vi "LoginVI.vi"() -> ()   [LabVIEW 2017]
uses:
  NameSurnameID.vi
panel:
  in  "Login information":T1
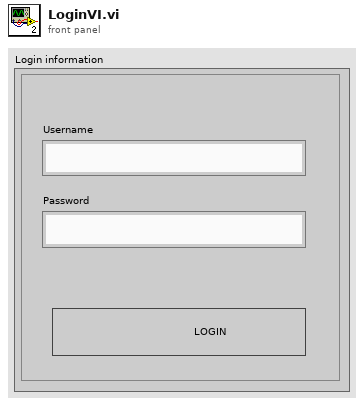
[diagram p1: front panel]
types:
  T1 = cluster{"Username":string, "Password":string, "Login button":bool}
  T2 = enum32{"Invalid", "Standard", "Closed", "Hidden", "Minimized", "Maximized"}
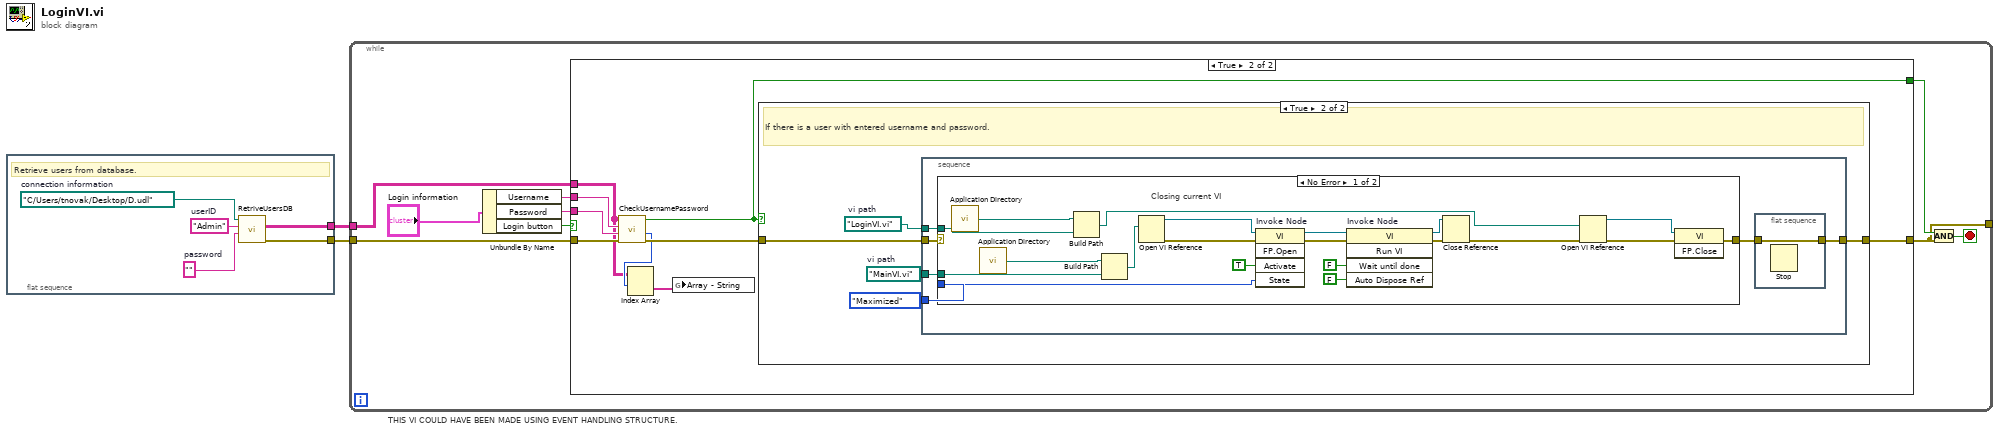
[diagram p0: block diagram]
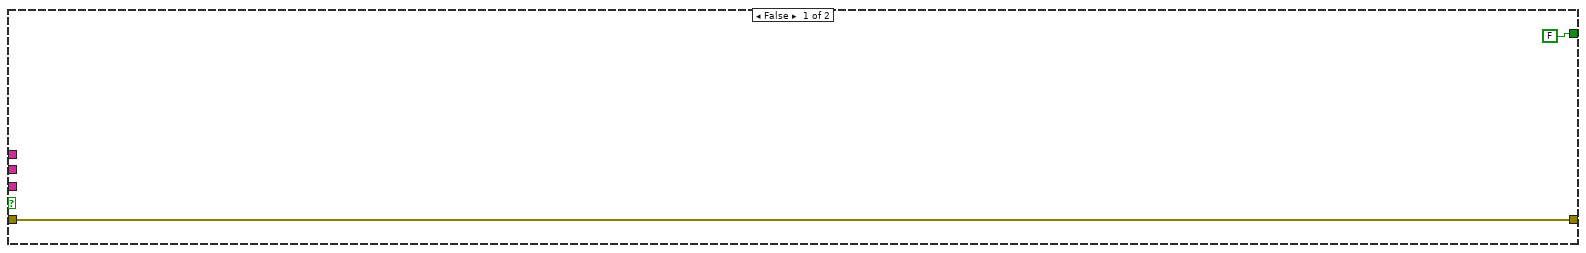
[diagram p2: hidden frame]
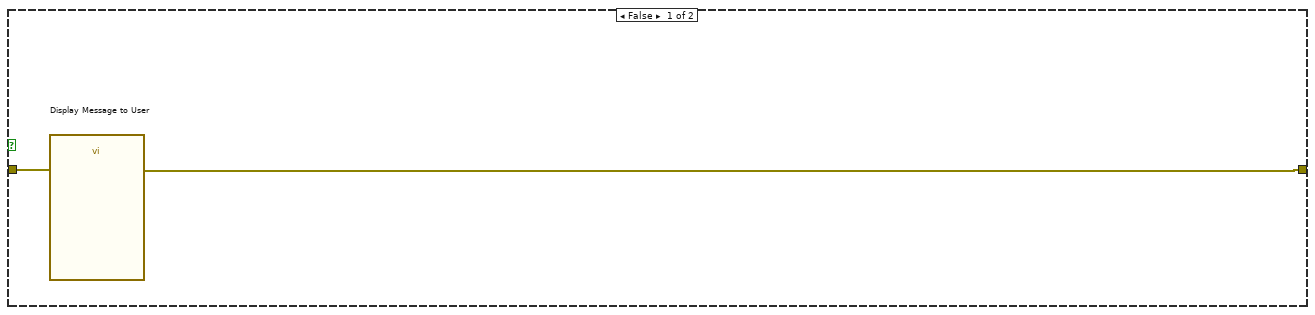
[diagram p3: hidden frame]
diagram:
  # "THIS VI COULD HAVE BEEN MADE USING EVENT HANDLING STRUCTURE."
  n1 = flat-sequence {
    tunnel: [w4] -> w2
    tunnel: [w3] -> w1
    frame #0 {
      w5 = ""  # password
      w6 = "Admin"  # userID
      w7 = path "C:/Users/tnovak/Desktop/D.udl"  # connection information
      # "Retrieve users from database."
      n2 = call "RetriveUsersDB.vi"("password"=w5, "userID"=w6, "connection information"=w7) -> ("error out"=w3:errorcluster, "Array"=w4:string[][])  [unwired: 7 in]
    }
  }
  n3 = while {
    tunnel: w2 -> [w12]
    tunnel: w1 -> [w11]
    tunnel: [w9] -> _
    stop <- w8 stop-if-true
    n4 = Unbundle By Name("Login information") -> ("Username"=w15:string, "Password"=w14:string, "Login button"=w13:bool)
    n5 = case shown="True" w13 {
      tunnel: w15 -> [_ w27]
      tunnel: w14 -> [_ w26]
      tunnel: w12 -> [_ w20]
      tunnel: w11 -> [w17 w24]
      tunnel: [FALSE w25] -> w10
      tunnel: [w17 w22] -> w9
      frame False {
      }
      frame True {
        n6 = call "CheckUsernamePassword.vi"("error in (no error)"=w24, "Password"=w26, "Username"=w27, "Array"=w20) -> ("error out"=w23:errorcluster, "Index of user"=w21:i32, "User exists"=w25:bool)  [unwired: 5 in]
        n7 = Index Array(array=w20, index (row)=w21) -> (element=w19:string[])  [unwired: 1 in]
        n8 = global write "NameSurnameID.vi" "Array - String"(w19) -> ()
        n9 = case shown="True" w25 {
          tunnel: [w28 w31] -> w22
          tunnel: w23 -> [w29 w32]
          frame False {
            n10 = call "Display Message to User"("error in (no error)"=w29) -> ("error out"=w28:errorcluster)  [unwired: 9 in, 1 out]
          }
          frame True {
            w30 = path "LoginVI.vi"  # vi path
            w33 = path "MainVI.vi"  # vi path
            # "If there is a user with entered username and password."
            n11 = stacked-sequence {
              tunnel: [w36] -> w31
              tunnel: w32 -> [w40]
              tunnel: T2."Maximized" ("State") -> [w39]
              tunnel: w33 -> [w38]
              tunnel: w30 -> [w35]
              frame #0 {
                n12 = case shown="No Error" w40 {
                  selector: w40 -> [_ w62]
                  tunnel: [w46 w62] -> w37
                  tunnel: w38 -> [w60 _]
                  tunnel: w39 -> [w52 _]
                  tunnel: w35 -> [w44 _]
                  frame No Error {
                    # "Closing current VI"
                    n13 = call <vilib>:"Application Directory.vi"() -> ("Application Directory"=w45:path)
                    n14 = call <vilib>:"Application Directory.vi"() -> ("Application Directory"=w59:path)
                    n15 = Build Path(base path=w45, name or relative path=w44) -> (appended path=w42:path)
                    n16 = Build Path(base path=w59, name or relative path=w60) -> (appended path=w61:path)
                    n17 = Open VI Reference(vi path=w61) -> (vi reference=w49:refnum<vi>, error out=w50:errorcluster)  [unwired: 1 in, 4 out]
                    n18 = invoke on="Invoke Node" class="VI" method="FP.Open"(reference=w49, error in=w50, "Activate"=TRUE ("Activate?"), "State"=w52) -> (reference out=w53:refnum<vi>, error out=w54:errorcluster)  [unwired: 1 in, 3 out]
                    n19 = invoke on="Invoke Node" class="VI" method="Run VI"(reference=w53, error in=w54, "Wait until done"=FALSE ("Wait Until Done"), "Auto Dispose Ref"=FALSE ("Auto Dispose Reference")) -> (reference out=w57:refnum<vi>, error out=w58:errorcluster)  [unwired: 1 in, 3 out]
                    n20 = Close Reference(reference=w57, error in (no error)=w58) -> (error out=w43:errorcluster)
                    n21 = Open VI Reference(vi path=w42, error in (no error)=w43) -> (vi reference=w48:refnum<vi>, error out=w47:errorcluster)  [unwired: 4 out]
                    n22 = invoke class="VI" method="FP.Close"(reference=w48, error in=w47) -> (error out=w46:errorcluster)  [unwired: 1 in, 2 out]
                  }
                  frame Error {
                  }
                }
                n23 = flat-sequence {
                  tunnel: w37 -> [w41]
                  tunnel: [w41] -> w36
                  frame #0 {
                    n24 = Stop() -> ()  [unwired: 1 in]
                  }
                }
              }
            }
          }
        }
      }
    }
    n25 = And(x=w10, y=w9) -> (x .and. y?=w8:bool)
  }
